vi "nanocal -- nuclear schottky fit V8.vi"() -> ()   [LabVIEW 2021] (continued)
 0.000000000000   ,  \"Reoff\" -> 0.000000000000   ,  \"Imoff\" -> 0.000000000000   ,  \"στ1\" -> 0.000000000000   ,  \"στS\" -> 0.000000000000   ,  \"στN\" -> 0.000000000000   ,  \"τ11 \" -> 0.000000000000   ,  \"τ12\" -> 0.000000000000   ,  \"τ22\" -> 0.000000000000   ,  \"τN1\" -> 0.000000000000   ,  \"τN2\" -> 0.000000000000   ,  \"σηlogτ1 \" -> 0.000000000000   ,  \"σηlogτS\" -> 0.000000000000   ,  \"σηlogτN\" -> 0.000000000000   ,  \"σlogτ1\" -> 0.000000000000   ,  \"σlogτS\" -> 0.000000000000   ,  \"σlogτN\" -> 0.000000000000   ,  \"σητ1\" -> 0.000000000000   ,  \"σητS \" -> 0.000000000000   ,  \"σητN\" -> 0.000000000000    |>   , \n\"IDS0168_210310_RAW_cal__ref_\" ->   <|    \"ζ\" -> 0.018175201883   ,  \"τ1\" -> 0.013383195137   ,  \"τS\" -> 0.017675939869   ,  \"τN\" -> 0.000584160710   ,  \"τC\" -> 0.005568397021   ,  \"κ0\" -> 0.000000005579   ,  \"mm1\" -> 0.000076155273   ,  \"mm2\" -> 0.012686054664   ,  \"mm3\" -> 0.024781363815   ,  \"T\" -> 0.810000000000   ,  \"B\" -> 12.000000000000   ,  \"θ\" -> 0.000000000000   ,  \"Reoff\" -> 0.000000000000   ,  \"Imoff\" -> 0.000000000000   ,  \"στ1\" -> 0.000105801087   ,  \"στS\" -> 0.000001832616   ,  \"στN\" -> 0.000002314917   ,  \"τ11 \" -> 0.000000000000   ,  \"τ12\" -> 0.000000000000   ,  \"τ22\" -> 0.000000000000   ,  \"τN1\" -> 0.000000000000   ,  \"τN2\" -> 0.000000000000   ,  \"σηlogτ1 \" -> 0.050518101739   ,  \"σηlogτS\" -> 0.000100664856   ,  \"σηlogτN\" -> 0.045919539288   ,  \"σlogτ1\" -> 0.007905517739   ,  \"σlogτS\" -> 0.000103678550   ,  \"σlogτN\" -> 0.003962808035   ,  \"σητ1\" -> 0.000676093614   ,  \"σητS \" -> 0.000001779346   ,  \"σητN\" -> 0.000026824391    |>   , \n\"IDS0168_210310_RAW_cal__sam_\" ->   <|    \"ζ\" -> 0.017558473054   ,  \"τ1\" -> 0.014545104284   ,  \"τS\" -> 0.022979681288   ,  \"τN\" -> 0.000840829385   ,  \"τC\" -> 0.005228030240   ,  \"κ0\" -> 0.000000006068   ,  \"mm1\" -> 0.000073916527   ,  \"mm2\" -> 0.013750428362   ,  \"mm3\" -> 0.030187552103   ,  \"T\" -> 0.810000000000   ,  \"B\" -> 12.000000000000   ,  \"θ\" -> 0.000000000000   ,  \"Reoff\" -> 0.000000000000   ,  \"Imoff\" -> 0.000000000000   ,  \"στ1\" -> 0.000000000000   ,  \"στS\" -> 0.000000000000   ,  \"στN\" -> 0.000000000000   ,  \"τ11 \" -> 0.000000000000   ,  \"τ12\" -> 0.000000000000   ,  \"τ22\" -> 0.000000000000   ,  \"τN1\" -> 0.000000000000   ,  \"τN2\" -> 0.000000000000   ,  \"σηlogτ1 \" -> 0.000000000000   ,  \"σηlogτS\" -> 0.000000000000   ,  \"σηlogτN\" -> 0.000000000000   ,  \"σlogτ1\" -> 0.000000000000   ,  \"σlogτS\" -> 0.000000000000   ,  \"σlogτN\" -> 0.000000000000   ,  \"σητ1\" -> 0.000000000000   ,  \"σητS \" -> 0.000000000000   ,  \"σητN\" -> 0.000000000000    |>   , \n\"IDS0169_210310_RAW_cal__ref_\" ->   <|    \"ζ\" -> 0.019957179421   ,  \"τ1\" -> 0.013979356395   ,  \"τS\" -> 0.014979933171   ,  \"τN\" -> 0.000246381668   ,  \"τC\" -> 0.003917957379   ,  \"κ0\" -> 0.000000007787   ,  \"mm1\" -> 0.000061209589   ,  \"mm2\" -> 0.013393834195   ,  \"mm3\" -> 0.019972459127   ,  \"T\" -> 1.120000000000   ,  \"B\" -> 12.000000000000   ,  \"θ\" -> 0.000000000000   ,  \"Reoff\" -> -604081.632653061067   ,  \"Imoff\" -> 0.000000000000   ,  \"στ1\" -> 0.016865078301   ,  \"στS\" -> 0.000159497722   ,  \"στN\" -> 0.007867947468   ,  \"τ11 \" -> 0.000000000000   ,  \"τ12\" -> 0.000000000000   ,  \"τ22\" -> 0.000000000000   ,  \"τN1\" -> 0.000000000000   ,  \"τN2\" -> 0.000000000000   ,  \"σηlogτ1 \" -> 0.000000000000   ,  \"σηlogτS\" -> 0.000000000000   ,  \"σηlogτN\" -> 0.000000000000   ,  \"σlogτ1\" -> 0.000000000000   ,  \"σlogτS\" -> 0.000000000000   ,  \"σlogτN\" -> 0.000000000000   ,  \"σητ1\" -> 0.000000000000   ,  \"σητS \" -> 0.000000000000   ,  \"σητN\" -> 0.000000000000    |>   , \n\"IDS0169_210310_RAW_cal__sam_\" ->   <|    \"ζ\" -> 0.011916480594   ,  \"τ1\" -> 0.012551282481   ,  \"τS\" -> 0.018233218660   ,  \"τN\" -> 0.000345702746   ,  \"τC\" -> 0.004699451527   ,  \"κ0\" -> 0.000000008451   ,  \"mm1\" -> 0.000044190864   ,  \"mm2\" -> 0.012162820727   ,  \"mm3\" -> 0.023844039179   ,  \"T\" -> 1.120000000000   ,  \"B\" -> 12.000000000000   ,  \"θ\" -> 0.000000000000   ,  \"Reoff\" -> 0.000000000000   ,  \"Imoff\" -> 0.000000000000   ,  \"στ1\" -> 0.000000000000   ,  \"στS\" -> 0.000000000000   ,  \"στN\" -> 0.000000000000   ,  \"τ11 \" -> 0.000000000000   ,  \"τ12\" -> 0.000000000000   ,  \"τ22\" -> 0.000000000000   ,  \"τN1\" -> 0.000000000000   ,  \"τN2\" -> 0.000000000000   ,  \"σηlogτ1 \" -> 0.000000000000   ,  \"σηlogτS\" -> 0.000000000000   ,  \"σηlogτN\" -> 0.000000000000   ,  \"σlogτ1\" -> 0.000000000000   ,  \"σlogτS\" -> 0.000000000000   ,  \"σlogτN\" -> 0.000000000000   ,  \"σητ1\" -> 0.000000000000   ,  \"σητS \" -> 0.000000000000   ,  \"σητN\" -> 0.000000000000    |>   , \n\"IDS0170_210310_RAW_cal__ref_\" ->   <|    \"ζ\" -> 0.020917521423   ,  \"τ1\" -> 0.014571936752   ,  \"τS\" -> 0.010774968577   ,  \"τN\" -> 0.000062073801   ,  \"τC\" -> 0.003888097391   ,  \"κ0\" -> 0.000000012613   ,  \"mm1\" -> 0.000059093319   ,  \"mm2\" -> 0.013758745196   ,  \"mm3\" -> 0.015705922073   ,  \"T\" -> 1.800000000000   ,  \"B\" -> 12.000000000000   ,  \"θ\" -> 0.000000000000   ,  \"Reoff\" -> -530612.244897959054   ,  \"Imoff\" -> 0.000000000000   ,  \"στ1\" -> 0.055735786157   ,  \"στS\" -> 0.000157216248   ,  \"στN\" -> 0.024225134913   ,  \"τ11 \" -> 0.000000000000   ,  \"τ12\" -> 0.000000000000   ,  \"τ22\" -> 0.000000000000   ,  \"τN1\" -> 0.000000000000   ,  \"τN2\" -> 0.000000000000   ,  \"σηlogτ1 \" -> 0.000000000000   ,  \"σηlogτS\" -> 0.000000000000   ,  \"σηlogτN\" -> 0.000000000000   ,  \"σlogτ1\" -> 0.000000000000   ,  \"σlogτS\" -> 0.000000000000   ,  \"σlogτN\" -> 0.000000000000   ,  \"σητ1\" -> 0.000000000000   ,  \"σητS \" -> 0.000000000000   ,  \"σητN\" -> 0.000000000000    |>   , \n\"IDS0170_210310_RAW_cal__sam_\" ->   <|    \"ζ\" -> 0.012831327568   ,  \"τ1\" -> 0.013315909415   ,  \"τS\" -> 0.012590836847   ,  \"τN\" -> 0.000065003013   ,  \"τC\" -> 0.005276356243   ,  \"κ0\" -> 0.000000013610   ,  \"mm1\" -> 0.000047406274   ,  \"mm2\" -> 0.013137605540   ,  \"mm3\" -> 0.018225484932   ,  \"T\" -> 1.800000000000   ,  \"B\" -> 12.000000000000   ,  \"θ\" -> 0.000000000000   ,  \"Reoff\" -> 0.000000000000   ,  \"Imoff\" -> 0.000000000000   ,  \"στ1\" -> 0.000000000000   ,  \"στS\" -> 0.000000000000   ,  \"στN\" -> 0.000000000000   ,  \"τ11 \" -> 0.000000000000   ,  \"τ12\" -> 0.000000000000   ,  \"τ22\" -> 0.000000000000   ,  \"τN1\" -> 0.000000000000   ,  \"τN2\" -> 0.000000000000   ,  \"σηlogτ1 \" -> 0.000000000000   ,  \"σηlogτS\" -> 0.000000000000   ,  \"σηlogτN\" -> 0.000000000000   ,  \"σlogτ1\" -> 0.000000000000   ,  \"σlogτS\" -> 0.000000000000   ,  \"σlogτN\" -> 0.000000000000   ,  \"σητ1\" -> 0.000000000000   ,  \"σητS \" -> 0.000000000000   ,  \"σητN\" -> 0.000000000000    |>   , \n\"IDS0171_210310_RAW_cal__ref_\" ->   <|    \"ζ\" -> 0.017116647721   ,  \"τ1\" -> 0.014941878219   ,  \"τS\" -> 0.008392436112   ,  \"τN\" -> 0.000011747084   ,  \"τC\" -> 0.002803142231   ,  \"κ0\" -> 0.000000022439   ,  \"mm1\" -> 0.000035623333   ,  \"mm2\" -> 0.011267010418   ,  \"mm3\" -> 0.014990421338   ,  \"T\" -> 3.100000000000   ,  \"B\" -> 12.000000000000   ,  \"θ\" -> 0.000000000000   ,  \"Reoff\" -> -297959.183673469349   ,  \"Imoff\" -> 0.000000000000   ,  \"στ1\" -> 0.410303910661   ,  \"στS\" -> 0.000232255759   ,  \"στN\" -> 0.188003802712   ,  \"τ11 \" -> 0.000000000000   ,  \"τ12\" -> 0.000000000000   ,  \"τ22\" -> 0.000000000000   ,  \"τN1\" -> 0.000000000000   ,  \"τN2\" -> 0.000000000000   ,  \"σηlogτ1 \" -> 0.000000000000   ,  \"σηlogτS\" -> 0.000000000000   ,  \"σηlogτN\" -> 0.000000000000   ,  \"σlogτ1\" -> 0.000000000000   ,  \"σlogτS\" -> 0.000000000000   ,  \"σlogτN\" -> 0.000000000000   ,  \"σητ1\" -> 0.000000000000   ,  \"σητS \" -> 0.000000000000   ,  \"σητN\" -> 0.000000000000    |>   , \n\"IDS0171_210310_RAW_cal__sam_\" ->   <|    \"ζ\" -> 0.019774146838   ,  \"τ1\" -> 0.013257273421   ,  \"τS\" -> 0.007064131508   ,  \"τN\" -> 0.000028000819   ,  \"τC\" -> 0.006942241845   ,  \"κ0\" -> 0.000000023477   ,  \"mm1\" -> 0.000068886863   ,  \"mm2\" -> 0.012935419574   ,  \"mm3\" -> 0.014427582022   ,  \"T\" -> 3.100000000000   ,  \"B\" -> 12.000000000000   ,  \"θ\" -> 0.000000000000   ,  \"Reoff\" -> 0.000000000000   ,  \"Imoff\" -> 0.000000000000   ,  \"στ1\" -> 0.000000000000   ,  \"στS\" -> 0.000000000000   ,  \"στN\" -> 0.000000000000   ,  \"τ11 \" -> 0.000000000000   ,  \"τ12\" -> 0.000000000000   ,  \"τ22\" -> 0.000000000000   ,  \"τN1\" -> 0.000000000000   ,  \"τN2\" -> 0.000000000000   ,  \"σηlogτ1 \" -> 0.000000000000   ,  \"σηlogτS\" -> 0.000000000000   ,  \"σηlogτN\" -> 0.000000000000   ,  \"σlogτ1\" -> 0.000000000000   ,  \"σlogτS\" -> 0.000000000000   ,  \"σlogτN\" -> 0.000000000000   ,  \"σητ1\" -> 0.000000000000   ,  \"σητS \" -> 0.000000000000   ,  \"σητN\" -> 0.000000000000    |>   , \n\"IDS0172_210310_RAW_cal__ref_\" ->   <|    \"ζ\" -> 0.018105234018   ,  \"τ1\" -> 0.013976020767   ,  \"τS\" -> 0.005494207082   ,  \"τN\" -> 0.000001697310   ,  \"τC\" -> 0.002434353238   ,  \"κ0\" -> 0.000000055294   ,  \"mm1\" -> 0.000030277813   ,  \"mm2\" -> 0.007995449956   ,  \"mm3\" -> 0.013980055263   ,  \"T\" -> 5.500000000000   ,  \"B\" -> 12.000000000000   ,  \"θ\" -> 0.000000000000   ,  \"Reoff\" -> -114285.714285714086   ,  \"Imoff\" -> 0.000000000000   ,  \"στ1\" -> 5.359406809289   ,  \"στS\" -> 0.000541837361   ,  \"στN\" -> 2.799281990955   ,  \"τ11 \" -> 0.000000000000   ,  \"τ12\" -> 0.000000000000   ,  \"τ22\" -> 0.000000000000   ,  \"τN1\" -> 0.000000000000   ,  \"τN2\" -> 0.000000000000   ,  \"σηlogτ1 \" -> 0.000000000000   ,  \"σηlogτS\" -> 0.000000000000   ,  \"σηlogτN\" -> 0.000000000000   ,  \"σlogτ1\" -> 0.000000000000   ,  \"σlogτS\" -> 0.000000000000   ,  \"σlogτN\" -> 0.000000000000   ,  \"σητ1\" -> 0.000000000000   ,  \"σητS \" -> 0.000000000000   ,  \"σητN\" -> 0.000000000000    |>   , \n\"IDS0172_210310_RAW_cal__sam_\" ->   <|    \"ζ\" -> 0.029251354442   ,  \"τ1\" -> 0.014634751206   ,  \"τS\" -> 0.003873958746   ,  \"τN\" -> 0.000007000487   ,  \"τC\" -> 0.006827504775   ,  \"κ0\" -> 0.000000056438   ,  \"mm1\" -> 0.000072018576   ,  \"mm2\" -> 0.010723236476   ,  \"mm3\" -> 0.014661483476   ,  \"T\" -> 5.500000000000   ,  \"B\" -> 12.000000000000   ,  \"θ\" -> 0.000000000000   ,  \"Reoff\" -> 0.000000000000   ,  \"Imoff\" -> 0.000000000000   ,  \"στ1\" -> 0.000000000000   ,  \"στS\" -> 0.000000000000   ,  \"στN\" -> 0.000000000000   ,  \"τ11 \" -> 0.000000000000   ,  \"τ12\" -> 0.000000000000   ,  \"τ22\" -> 0.000000000000   ,  \"τN1\" -> 0.000000000000   ,  \"τN2\" -> 0.000000000000   ,  \"σηlogτ1 \" -> 0.000000000000   ,  \"σηlogτS\" -> 0.000000000000   ,  \"σηlogτN\" -> 0.000000000000   ,  \"σlogτ1\" -> 0.000000000000   ,  \"σlogτS\" -> 0.000000000000   ,  \"σlogτN\" -> 0.000000000000   ,  \"σητ1\" -> 0.000000000000   ,  \"σητS \" -> 0.000000000000   ,  \"σητN\" -> 0.000000000000    |>   , \n\"IDS0181_210310_RAW_cal__ref_\" ->   <|    \"ζ\" -> 0.199306617611   ,  \"τ1\" -> 0.070107577087   ,  \"τS\" -> 0.034354681127   ,  \"τN\" -> 0.115326183519   ,  \"τC\" -> 0.001029913549   ,  \"κ0\" -> 0.000000000906   ,  \"mm1\" -> 0.000167619565   ,  \"mm2\" -> 0.012387908692   ,  \"mm3\" -> 0.238095213878   ,  \"T\" -> 0.179000000000   ,  \"B\" -> 12.000000000000   ,  \"θ\" -> 90.000000000000   ,  \"Reoff\" -> 0.000000000000   ,  \"Imoff\" -> 0.000000000000   ,  \"στ1\" -> 0.000080290810   ,  \"στS\" -> 0.000013361577   ,  \"στN\" -> 0.000100930245   ,  \"τ11 \" -> 0.000000000000   ,  \"τ12\" -> 0.000000000000   ,  \"τ22\" -> 0.000000000000   ,  \"τN1\" -> 0.000000000000   ,  \"τN2\" -> 0.000000000000   ,  \"σηlogτ1 \" -> 0.034187158287   ,  \"σηlogτS\" -> 0.001052177546   ,  \"σηlogτN\" -> 0.047354437967   ,  \"σlogτ1\" -> 0.001145251526   ,  \"σlogτS\" -> 0.000388930305   ,  \"σlogτN\" -> 0.000875171988   ,  \"σητ1\" -> 0.002396778835   ,  \"σητS \" -> 0.000036147224   ,  \"σητN\" -> 0.005461206603    |>   , \n\"IDS0181_210310_RAW_cal__sam_\" ->   <|    \"ζ\" -> 0.161975781729   ,  \"τ1\" -> 0.073089805113   ,  \"τS\" -> 0.045018408115   ,  \"τN\" -> 0.161987434028   ,  \"τC\" -> 0.001482104484   ,  \"κ0\" -> 0.000000001038   ,  \"mm1\" -> 0.000201615809   ,  \"mm2\" -> 0.012976126678   ,  \"mm3\" -> 0.301929942357   ,  \"T\" -> 0.179000000000   ,  \"B\" -> 12.000000000000   ,  \"θ\" -> 90.000000000000   ,  \"Reoff\" -> 0.000000000000   ,  \"Imoff\" -> 0.000000000000   ,  \"στ1\" -> 0.000000000000   ,  \"στS\" -> 0.000000000000   ,  \"στN\" -> 0.000000000000   ,  \"τ11 \" -> 0.000000000000   ,  \"τ12\" -> 0.000000000000   ,  \"τ22\" -> 0.000000000000   ,  \"τN1\" -> 0.000000000000   ,  \"τN2\" -> 0.000000000000   ,  \"σηlogτ1 \" -> 0.000000000000   ,  \"σηlogτS\" -> 0.000000000000   ,  \"σηlogτN\" -> 0.000000000000   ,  \"σlogτ1\" -> 0.000000000000   ,  \"σlogτS\" -> 0.000000000000   ,  \"σlogτN\" -> 0.000000000000   ,  \"σητ1\" -> 0.000000000000   ,  \"σητS \" -> 0.000000000000   ,  \"σητN\" -> 0.000000000000    |>   , \n\"IDS0183_210310_RAW_cal__ref_\" ->   <|    \"ζ\" -> 0.375235391174   ,  \"τ1\" -> 0.100390183494   ,  \"τS\" -> 0.059883674441   ,  \"τN\" -> 0.583268417564   ,  \"τC\" -> 0.001015388210   ,  \"κ0\" -> 0.000000000451   ,  \"mm1\" -> 0.000274513115   ,  \"mm2\" -> 0.008539722831   ,  \"mm3\" -> 0.977076854592   ,  \"T\" -> 0.120000000000   ,  \"B\" -> 12.000000000000   ,  \"θ\" -> 90.000000000000   ,  \"Reoff\" -> 0.000000000000   ,  \"Imoff\" -> 0.000000000000   ,  \"στ1\" -> 0.000375271363   ,  \"στS\" -> 0.000128650872   ,  \"στN\" -> 0.001598463820   ,  \"τ11 \" -> 0.000000000000   ,  \"τ12\" -> 0.000000000000   ,  \"τ22\" -> 0.000000000000   ,  \"τN1\" -> 0.000000000000   ,  \"τN2\" -> 0.000000000000   ,  \"σηlogτ1 \" -> 0.048375297950   ,  \"σηlogτS\" -> 0.002019546500   ,  \"σηlogτN\" -> 0.062171656813   ,  \"σlogτ1\" -> 0.003738128067   ,  \"σlogτS\" -> 0.002148346326   ,  \"σlogτN\" -> 0.002740528669   ,  \"σητ1\" -> 0.004856405038   ,  \"σητS \" -> 0.000120937865   ,  \"σητN\" -> 0.036262763887    |>   , \n\"IDS0183_210310_RAW_cal__sam_\" ->   <|    \"ζ\" -> 0.300863384227   ,  \"τ1\" -> 0.104924004009   ,  \"τS\" -> 0.071070599729   ,  \"τN\" -> 0.992887187112   ,  \"τC\" -> 0.001721587800   ,  \"κ0\" -> 0.000000000548   ,  \"mm1\" -> 0.000392216822   ,  \"mm2\" -> 0.006637384427   ,  \"mm3\" -> 1.483679717825   ,  \"T\" -> 0.120000000000   ,  \"B\" -> 12.000000000000   ,  \"θ\" -> 90.000000000000   ,  \"Reoff\" -> 0.000000000000   ,  \"Imoff\" -> 0.000000000000   ,  \"στ1\" -> 0.000000000000   ,  \"στS\" -> 0.000000000000   ,  \"στN\" -> 0.000000000000   ,  \"τ11 \" -> 0.000000000000   ,  \"τ12\" -> 0.000000000000   ,  \"τ22\" -> 0.000000000000   ,  \"τN1\" -> 0.000000000000   ,  \"τN2\" -> 0.000000000000   ,  \"σηlogτ1 \" -> 0.000000000000   ,  \"σηlogτS\" -> 0.000000000000   ,  \"σηlogτN\" -> 0.000000000000   ,  \"σlogτ1\" -> 0.000000000000   ,  \"σlogτS\" -> 0.000000000000   ,  \"σlogτN\" -> 0.000000000000   ,  \"σητ1\" -> 0.000000000000   ,  \"σητS \" -> 0.000000000000   ,  \"σητN\" -> 0.000000000000    |>   , \n\"IDS0184_210310_RAW_cal__ref_\" ->   <|    \"ζ\" -> 0.267189614091   ,  \"τ1\" -> 0.086925369127   ,  \"τS\" -> 0.044416499058   ,  \"τN\" -> 0.254096954422   ,  \"τC\" -> 0.000963914391   ,  \"κ0\" -> 0.000000000659   ,  \"mm1\" -> 0.000200487571   ,  \"mm2\" -> 0.010899085515   ,  \"mm3\" -> 0.455062858348   ,  \"T\" -> 0.148000000000   ,  \"B\" -> 12.000000000000   ,  \"θ\" -> 90.000000000000   ,  \"Reoff\" -> 0.000000000000   ,  \"Imoff\" -> 0.000000000000   ,  \"στ1\" -> 0.000162673595   ,  \"στS\" -> 0.000036959811   ,  \"στN\" -> 0.000362772077   ,  \"τ11 \" -> 0.000000000000   ,  \"τ12\" -> 0.000000000000   ,  \"τ22\" -> 0.000000000000   ,  \"τN1\" -> 0.000000000000   ,  \"τN2\" -> 0.000000000000   ,  \"σηlogτ1 \" -> 0.039106583663   ,  \"σηlogτS\" -> 0.001480745607   ,  \"σηlogτN\" -> 0.052582206660   ,  \"σlogτ1\" -> 0.001871416790   ,  \"σlogτS\" -> 0.000832118957   ,  \"σlogτN\" -> 0.001427691560   ,  \"σητ1\" -> 0.003399354220   ,  \"σητS \" -> 0.000065769536   ,  \"σητN\" -> 0.013360978569    |>   , \n\"IDS0184_210310_RAW_cal__sam_\" ->   <|    \"ζ\" -> 0.215697702358   ,  \"τ1\" -> 0.095971807771   ,  \"τS\" -> 0.069319630290   ,  \"τN\" -> 0.366712218878   ,  \"τC\" -> 0.001526252261   ,  \"κ0\" -> 0.000000000784   ,  \"mm1\" -> 0.000266752031   ,  \"mm2\" -> 0.013373263674   ,  \"mm3\" -> 0.613940961515   ,  \"T\" -> 0.148000000000   ,  \"B\" -> 12.000000000000   ,  \"θ\" -> 90.000000000000   ,  \"Reoff\" -> 0.000000000000   ,  \"Imoff\" -> 0.000000000000   ,  \"στ1\" -> 0.000000000000   ,  \"στS\" -> 0.000000000000   ,  \"στN\" -> 0.000000000000   ,  \"τ11 \" -> 0.000000000000   ,  \"τ12\" -> 0.000000000000   ,  \"τ22\" -> 0.000000000000   ,  \"τN1\" -> 0.000000000000   ,  \"τN2\" -> 0.000000000000   ,  \"σηlogτ1 \" -> 0.000000000000   ,  \"σηlogτS\" -> 0.000000000000   ,  \"σηlogτN\" -> 0.000000000000   ,  \"σlogτ1\" -> 0.000000000000   ,  \"σlogτS\" -> 0.000000000000   ,  \"σlogτN\" -> 0.000000000000   ,  \"σητ1\" -> 0.000000000000   ,  \"σητS \" -> 0.000000000000   ,  \"σητN\" -> 0.000000000000    |>   , \n\"IDS0185_210310_RAW_cal__ref_\" ->   <|    \"ζ\" -> 0.169435500052   ,  \"τ1\" -> 0.065522222520   ,  \"τS\" -> 0.031885966152   ,  \"τN\" -> 0.085736532349   ,  \"τC\" -> 0.001085511850   ,  \"κ0\" -> 0.000000001071   ,  \"mm1\" -> 0.000153416807   ,  \"mm2\" -> 0.013121484947   ,  \"mm3\" -> 0.190884757967   ,  \"T\" -> 0.197000000000   ,  \"B\" -> 12.000000000000   ,  \"θ\" -> 90.000000000000   ,  \"Reoff\" -> 0.000000000000   ,  \"Imoff\" -> 0.000000000000   ,  \"στ1\" -> 0.000057538627   ,  \"στS\" -> 0.000008322484   ,  \"στN\" -> 0.000057382706   ,  \"τ11 \" -> 0.000000000000   ,  \"τ12\" -> 0.000000000000   ,  \"τ22\" -> 0.000000000000   ,  \"τN1\" -> 0.000000000000   ,  \"τN2\" -> 0.000000000000   ,  \"σηlogτ1 \" -> 0.032785245148   ,  \"σηlogτS\" -> 0.000886609066   ,  \"σηlogτN\" -> 0.045894988103   ,  \"σlogτ1\" -> 0.000878154381   ,  \"σlogτS\" -> 0.000261007731   ,  \"σlogτN\" -> 0.000669291195   ,  \"σητ1\" -> 0.002148162128   ,  \"σητS \" -> 0.000028270387   ,  \"σητN\" -> 0.003934877132    |>   , \n\"IDS0185_210310_RAW_cal__sam_\" ->   <|    \"ζ\" -> 0.139117463690   ,  \"τ1\" -> 0.070330410174   ,  \"τS\" -> 0.040829719954   ,  \"τN\" -> 0.122434321115   ,  \"τC\" -> 0.001436112939   ,  \"κ0\" -> 0.000000001208   ,  \"mm1\" -> 0.000170710071   ,  \"mm2\" -> 0.013785404893   ,  \"mm3\" -> 0.243787328523   ,  \"T\" -> 0.197000000000   ,  \"B\" -> 12.000000000000   ,  \"θ\" -> 90.000000000000   ,  \"Reoff\" -> 0.000000000000   ,  \"Imoff\" -> 0.000000000000   ,  \"στ1\" -> 0.000000000000   ,  \"στS\" -> 0.000000000000   ,  \"στN\" -> 0.000000000000   ,  \"τ11 \" -> 0.000000000000   ,  \"τ12\" -> 0.000000000000   ,  \"τ22\" -> 0.000000000000   ,  \"τN1\" -> 0.000000000000   ,  \"τN2\" -> 0.000000000000   ,  \"σηlogτ1 \" -> 0.000000000000   ,  \"σηlogτS\" -> 0.000000000000   ,  \"σηlogτN\" -> 0.000000000000   ,  \"σlogτ1\" -> 0.000000000000   ,  \"σlogτS\" -> 0.000000000000   ,  \"σlogτN\" -> 0.000000000000   ,  \"σητ1\" -> 0.000000000000   ,  \"σητS \" -> 0.000000000000   ,  \"σητN\" -> 0.000000000000    |>   , \n\"IDS0186_210310_RAW_cal__ref_\" ->   <|    \"ζ\" -> 0.100232193660   ,  \"τ1\" -> 0.049981714900   ,  \"τS\" -> 0.026964705596   ,  \"τN\" -> 0.034498560244   ,  \"τC\" -> 0.001422553924   ,  \"κ0\" -> 0.000000001370   ,  \"mm1\" -> 0.000124145367   ,  \"mm2\" -> 0.014880634319   ,  \"mm3\" -> 0.104023352943   ,  \"T\" -> 0.249000000000   ,  \"B\" -> 12.000000000000   ,  \"θ\" -> 90.000000000000   ,  \"Reoff\" -> 0.000000000000   ,  \"Imoff\" -> 0.000000000000   ,  \"στ1\" -> 0.000091233173   ,  \"στS\" -> 0.000009463067   ,  \"στN\" -> 0.000045871847   ,  \"τ11 \" -> 0.000000000000   ,  \"τ12\" -> 0.000000000000   ,  \"τ22\" -> 0.000000000000   ,  \"τN1\" -> 0.000000000000   ,  \"τN2\" -> 0.000000000000   ,  \"σηlogτ1 \" -> 0.031503726160   ,  \"σηlogτS\" -> 0.000569534267   ,  \"σηlogτN\" -> 0.043675133431   ,  \"σlogτ1\" -> 0.001825330990   ,  \"σlogτS\" -> 0.000350942719   ,  \"σlogτN\" -> 0.001329674256   ,  \"σητ1\" -> 0.001574610259   ,  \"σητS \" -> 0.000015357324   ,  \"σητN\" -> 0.001506729222    |>   , \n\"IDS0186_210310_RAW_cal__sam_\" ->   <|    \"ζ\" -> 0.079912790251   ,  \"τ1\" -> 0.053932962768   ,  \"τS\" -> 0.033847624645   ,  \"τN\" -> 0.047947649984   ,  \"τC\" -> 0.001828917906   ,  \"κ0\" -> 0.000000001546   ,  \"mm1\" -> 0.000129305669   ,  \"mm2\" -> 0.016142481427   ,  \"mm3\" -> 0.127821856832   ,  \"T\" -> 0.249000000000   ,  \"B\" -> 12.000000000000   ,  \"θ\" -> 90.000000000000   ,  \"Reoff\" -> 0.000000000000   ,  \"Imoff\" -> 0.000000000000   ,  \"στ1\" -> 0.000000000000   ,  \"στS\" -> 0.000000000000   ,  \"στN\" -> 0.000000000000   ,  \"τ11 \" -> 0.000000000000   ,  \"τ12\" -> 0.000000000000   ,  \"τ22\" -> 0.000000000000   ,  \"τN1\" -> 0.000000000000   ,  \"τN2\" -> 0.000000000000   ,  \"σηlogτ1 \" -> 0.000000000000   ,  \"σηlogτS\" -> 0.000000000000   ,  \"σηlogτN\" -> 0.000000000000   ,  \"σlogτ1\" -> 0.000000000000   ,  \"σlogτS\" -> 0.000000000000   ,  \"σlogτN\" -> 0.000000000000   ,  \"σητ1\" -> 0.000000000000   ,  \"σητS \" -> 0.000000000000   ,  \"σητN\" -> 0.000000000000    |>   , \n\"IDS0187_210310_RAW_cal__ref_\" ->   <|    \"ζ\" -> 0.068889386962   ,  \"τ1\" -> 0.042189760597   ,  \"τS\" -> 0.023837806105   ,  \"τN\" -> 0.017176281362   ,  \"τC\" -> 0.001657645209   ,  \"κ0\" -> 0.000000001746   ,  \"mm1\" -> 0.000100672139   ,  \"mm2\" -> 0.015917651868   ,  \"mm3\" -> 0.071668604609   ,  \"T\" -> 0.300000000000   ,  \"B\" -> 12.000000000000   ,  \"θ\" -> 90.000000000000   ,  \"Reoff\" -> 0.000000000000   ,  \"Imoff\" -> 0.000000000000   ,  \"στ1\" -> 0.000071502532   ,  \"στS\" -> 0.000005082442   ,  \"στN\" -> 0.000020526312   ,  \"τ11 \" -> 0.000000000000   ,  \"τ12\" -> 0.000000000000   ,  \"τ22\" -> 0.000000000000   ,  \"τN1\" -> 0.000000000000   ,  \"τN2\" -> 0.000000000000   ,  \"σηlogτ1 \" -> 0.031154246719   ,  \"σηlogτS\" -> 0.000371188322   ,  \"σηlogτN\" -> 0.042807799707   ,  \"σlogτ1\" -> 0.001694784024   ,  \"σlogτS\" -> 0.000213209307   ,  \"σlogτN\" -> 0.001195038160   ,  \"σητ1\" -> 0.001314390211   ,  \"σητS \" -> 0.000008848315   ,  \"σητN\" -> 0.000735278812    |>   , \n\"IDS0187_210310_RAW_cal__sam_\" ->   <|    \"ζ\" -> 0.057938569833   ,  \"τ1\" -> 0.045244527663   ,  \"τS\" -> 0.029709028064   ,  \"τN\" -> 0.023577376257   ,  \"τC\" -> 0.002006607539   ,  \"κ0\" -> 0.000000001948   ,  \"mm1\" -> 0.000103608352   ,  \"mm2\" -> 0.017542867394   ,  \"mm3\" -> 0.085978401835   ,  \"T\" -> 0.300000000000   ,  \"B\" -> 12.000000000000   ,  \"θ\" -> 90.000000000000   ,  \"Reoff\" -> 0.000000000000   ,  \"Imoff\" -> 0.000000000000   ,  \"στ1\" -> 0.000000000000   ,  \"στS\" -> 0.000000000000   ,  \"στN\" -> 0.000000000000   ,  \"τ11 \" -> 0.000000000000   ,  \"τ12\" -> 0.000000000000   ,  \"τ22\" -> 0.000000000000   ,  \"τN1\" -> 0.000000000000   ,  \"τN2\" -> 0.000000000000   ,  \"σηlogτ1 \" -> 0.000000000000   ,  \"σηlogτS\" -> 0.000000000000   ,  \"σηlogτN\" -> 0.000000000000   ,  \"σlogτ1\" -> 0.000000000000   ,  \"σlogτS\" -> 0.000000000000   ,  \"σlogτN\" -> 0.000000000000   ,  \"σητ1\" -> 0.000000000000   ,  \"σητS \" -> 0.000000000000   ,  \"σητN\" -> 0.000000000000    |>   , \n\"IDS0188_210310_RAW_cal__ref_\" ->   <|    \"ζ\" -> 0.050855621628   ,  \"τ1\" -> 0.035114064267   ,  \"τS\" -> 0.021745076003   ,  \"τN\" -> 0.009940720882   ,  \"τC\" -> 0.002035754152   ,  \"κ0\" -> 0.000000002124   ,  \"mm1\" -> 0.000090783062   ,  \"mm2\" -> 0.016027821307   ,  \"mm3\" -> 0.054328411833   ,  \"T\" -> 0.360000000000   ,  \"B\" -> 12.000000000000   ,  \"θ\" -> 90.000000000000   ,  \"Reoff\" -> 0.000000000000   ,  \"Imoff\" -> 0.000000000000   ,  \"στ1\" -> 0.000051164040   ,  \"στS\" -> 0.000002904884   ,  \"στN\" -> 0.000009775078   ,  \"τ11 \" -> 0.000000000000   ,  \"τ12\" -> 0.000000000000   ,  \"τ22\" -> 0.000000000000   ,  \"τN1\" -> 0.000000000000   ,  \"τN2\" -> 0.000000000000   ,  \"σηlogτ1 \" -> 0.032086752475   ,  \"σηlogτS\" -> 0.000290620320   ,  \"σηlogτN\" -> 0.042734154502   ,  \"σlogτ1\" -> 0.001457081108   ,  \"σlogτS\" -> 0.000133588143   ,  \"σlogτN\" -> 0.000983336979   ,  \"σητ1\" -> 0.001126696289   ,  \"σητS \" -> 0.000006319561   ,  \"σητN\" -> 0.000424808302    |>   , \n\"IDS0188_210310_RAW_cal__sam_\" ->   <|    \"ζ\" -> 0.044154556051   ,  \"τ1\" -> 0.038823125235   ,  \"τS\" -> 0.027069314930   ,  \"τN\" -> 0.013601990730   ,  \"τC\" -> 0.002287979276   ,  \"κ0\" -> 0.000000002359   ,  \"mm1\" -> 0.000089763345   ,  \"mm2\" -> 0.018083678254   ,  \"mm3\" -> 0.065404792018   ,  \"T\" -> 0.360000000000   ,  \"B\" -> 12.000000000000   ,  \"θ\" -> 90.000000000000   ,  \"Reoff\" -> 0.000000000000   ,  \"Imoff\" -> 0.000000000000   ,  \"στ1\" -> 0.000000000000   ,  \"στS\" -> 0.000000000000   ,  \"στN\" -> 0.000000000000   ,  \"τ11 \" -> 0.000000000000   ,  \"τ12\" -> 0.000000000000   ,  \"τ22\" -> 0.000000000000   ,  \"τN1\" -> 0.000000000000   ,  \"τN2\" -> 0.000000000000   ,  \"σηlogτ1 \" -> 0.000000000000   ,  \"σηlogτS\" -> 0.000000000000   ,  \"σηlogτN\" -> 0.000000000000   ,  \"σlogτ1\" -> 0.000000000000   ,  \"σlogτS\" -> 0.000000000000   ,  \"σlogτN\" -> 0.000000000000   ,  \"σητ1\" -> 0.000000000000   ,  \"σητS \" -> 0.000000000000   ,  \"σητN\" -> 0.000000000000    |>   , \n\"IDS0189_210310_RAW_cal__ref_\" ->   <|    \"ζ\" -> 0.038379394547   ,  \"τ1\" -> 0.030049345911   ,  \"τS\" -> 0.020197203084   ,  \"τN\" -> 0.005279271749   ,  \"τC\" -> 0.002296433055   ,  \"κ0\" -> 0.000000002676   ,  \"mm1\" -> 0.000076749631   ,  \"mm2\" -> 0.016510358322   ,  \"mm3\" -> 0.042212917525   ,  \"T\" -> 0.430000000000   ,  \"B\" -> 12.000000000000   ,  \"θ\" -> 90.000000000000   ,  \"Reoff\" -> 0.000000000000   ,  \"Imoff\" -> 0.000000000000   ,  \"στ1\" -> 0.000059898317   ,  \"στS\" -> 0.000002370734   ,  \"στN\" -> 0.000006802565   ,  \"τ11 \" -> 0.000000000000   ,  \"τ12\" -> 0.000000000000   ,  \"τ22\" -> 0.000000000000   ,  \"τN1\" -> 0.000000000000   ,  \"τN2\" -> 0.000000000000   ,  \"σηlogτ1 \" -> 0.033097505686   ,  \"σηlogτS\" -> 0.000200297015   ,  \"σηlogτN\" -> 0.042720953668   ,  \"σlogτ1\" -> 0.001993331815   ,  \"σlogτS\" -> 0.000117379325   ,  \"σlogτN\" -> 0.001288542279   ,  \"σητ1\" -> 0.000994558397   ,  \"σητS \" -> 0.000004045439   ,  \"σητN\" -> 0.000225535524    |>   , \n\"IDS0189_210310_RAW_cal__sam_\" ->   <|    \"ζ\" -> 0.032748569996   ,  \"τ1\" -> 0.031072007290   ,  \"τS\" -> 0.024343937548   ,  \"τN\" -> 0.006961654481   ,  \"τC\" -> 0.002967111565   ,  \"κ0\" -> 0.000000002964   ,  \"mm1\" -> 0.000084402249   ,  \"mm2\" -> 0.018055855929   ,  \"mm3\" -> 0.048229666078   ,  \"T\" -> 0.430000000000   ,  \"B\" -> 12.000000000000   ,  \"θ\" -> 90.000000000000   ,  \"Reoff\" -> 0.000000000000   ,  \"Imoff\" -> 0.000000000000   ,  \"στ1\" -> 0.000000000000   ,  \"στS\" -> 0.000000000000   ,  \"στN\" -> 0.000000000000   ,  \"τ11 \" -> 0.000000000000   ,  \"τ12\" -> 0.000000000000   ,  \"τ22\" -> 0.000000000000   ,  \"τN1\" -> 0.000000000000   ,  \"τN2\" -> 0.000000000000   ,  \"σηlogτ1 \" -> 0.000000000000   ,  \"σηlogτS\" -> 0.000000000000   ,  \"σηlogτN\" -> 0.000000000000   ,  \"σlogτ1\" -> 0.000000000000   ,  \"σlogτS\" -> 0.000000000000   ,  \"σlogτN\" -> 0.000000000000   ,  \"σητ1\" -> 0.000000000000   ,  \"σητS \" -> 0.000000000000   ,  \"σητN\" -> 0.000000000000    |>   , \n\"IDS0190_210310_RAW_cal__ref_\" ->   <|    \"ζ\" -> 0.030757711173   ,  \"τ1\" -> 0.024931554661   ,  \"τS\" -> 0.019059366283   ,  \"τN\" -> 0.002804912424   ,  \"τC\" -> 0.002400955690   ,  \"κ0\" -> 0.000000003344   ,  \"mm1\" -> 0.000064025305   ,  \"mm2\" -> 0.016413784329   ,  \"mm3\" -> 0.033391474593   ,  \"T\" -> 0.512000000000   ,  \"B\" -> 12.000000000000   ,  \"θ\" -> 90.000000000000   ,  \"Reoff\" -> 0.000000000000   ,  \"Imoff\" -> 0.000000000000   ,  \"στ1\" -> 0.000088127283   ,  \"στS\" -> 0.000002533160   ,  \"στN\" -> 0.000006068263   ,  \"τ11 \" -> 0.000000000000   ,  \"τ12\" -> 0.000000000000   ,  \"τ22\" -> 0.000000000000   ,  \"τN1\" -> 0.000000000000   ,  \"τN2\" -> 0.000000000000   ,  \"σηlogτ1 \" -> 0.035038614150   ,  \"σηlogτS\" -> 0.000144373831   ,  \"σηlogτN\" -> 0.043033459724   ,  \"σlogτ1\" -> 0.003534768852   ,  \"σlogτS\" -> 0.000132908910   ,  \"σlogτN\" -> 0.002163441144   ,  \"σητ1\" -> 0.000873567124   ,  \"σητS \" -> 0.000002751674   ,  \"σητN\" -> 0.000120705086    |>   , \n\"IDS0190_210310_RAW_cal__sam_\" ->   <|    \"ζ\" -> 0.027599263457   ,  \"τ1\" -> 0.026239105728   ,  \"τS\" -> 0.022370859308   ,  \"τN\" -> 0.003857632966   ,  \"τC\" -> 0.003499360499   ,  \"κ0\" -> 0.000000003681   ,  \"mm1\" -> 0.000081816106   ,  \"mm2\" -> 0.017901054668   ,  \"mm3\" -> 0.038707974796   ,  \"T\" -> 0.512000000000   ,  \"B\" -> 12.000000000000   ,  \"θ\" -> 90.000000000000   ,  \"Reoff\" -> 0.000000000000   ,  \"Imoff\" -> 0.000000000000   ,  \"στ1\" -> 0.000000000000   ,  \"στS\" -> 0.000000000000   ,  \"στN\" -> 0.000000000000   ,  \"τ11 \" -> 0.000000000000   ,  \"τ12\" -> 0.000000000000   ,  \"τ22\" -> 0.000000000000   ,  \"τN1\" -> 0.000000000000   ,  \"τN2\" -> 0.000000000000   ,  \"σηlogτ1 \" -> 0.000000000000   ,  \"σηlogτS\" -> 0.000000000000   ,  \"σηlogτN\" -> 0.000000000000   ,  \"σlogτ1\" -> 0.000000000000   ,  \"σlogτS\" -> 0.000000000000   ,  \"σlogτN\" -> 0.000000000000   ,  \"σητ1\" -> 0.000000000000   ,  \"σητS \" -> 0.000000000000   ,  \"σητN\" -> 0.000000000000    |>   , \n\"IDS0191_210310_RAW_cal__ref_\" ->   <|    \"ζ\" -> 0.024472356387   ,  \"τ1\" -> 0.022407083343   ,  \"τS\" -> 0.017600386438   ,  \"τN\" -> 0.001730254025   ,  \"τC\" -> 0.003444856237   ,  \"κ0\" -> 0.000000003989   ,  \"mm1\" -> 0.000069310557   ,  \"mm2\" -> 0.016480900420   ,  \"mm3\" -> 0.029105435389   ,  \"T\" -> 0.610000000000   ,  \"B\" -> 12.000000000000   ,  \"θ\" -> 90.000000000000   ,  \"Reoff\" -> 0.000000000000   ,  \"Imoff\" -> 0.000000000000   ,  \"στ1\" -> 0.000087154359   ,  \"στS\" -> 0.000001846195   ,  \"στN\" -> 0.000003983538   ,  \"τ11 \" -> 0.000000000000   ,  \"τ12\" -> 0.000000000000   ,  \"τ22\" -> 0.000000000000   ,  \"τN1\" -> 0.000000000000   ,  \"τN2\" -> 0.000000000000   ,  \"σηlogτ1 \" -> 0.036359774839   ,  \"σηlogτS\" -> 0.000111954983   ,  \"σηlogτN\" -> 0.043247347257   ,  \"σlogτ1\" -> 0.003889589636   ,  \"σlogτS\" -> 0.000104895132   ,  \"σlogτN\" -> 0.002302284973   ,  \"σητ1\" -> 0.000814716505   ,  \"σητS \" -> 0.000001970451   ,  \"σητN\" -> 0.000074828897    |>   , \n\"IDS0191_210310_RAW_cal__sam_\" ->   <|    \"ζ\" -> 0.020568815513   ,  \"τ1\" -> 0.023045965648   ,  \"τS\" -> 0.020791387386   ,  \"τN\" -> 0.002229171297   ,  \"τC\" -> 0.004427475438   ,  \"κ0\" -> 0.000000004398   ,  \"mm1\" -> 0.000074037290   ,  \"mm2\" -> 0.017820522459   ,  \"mm3\" -> 0.033072945644   ,  \"T\" -> 0.610000000000   ,  \"B\" -> 12.000000000000   ,  \"θ\" -> 90.000000000000   ,  \"Reoff\" -> 0.000000000000   ,  \"Imoff\" -> 0.000000000000   ,  \"στ1\" -> 0.000000000000   ,  \"στS\" -> 0.000000000000   ,  \"στN\" -> 0.000000000000   ,  \"τ11 \" -> 0.000000000000   ,  \"τ12\" -> 0.000000000000   ,  \"τ22\" -> 0.000000000000   ,  \"τN1\" -> 0.000000000000   ,  \"τN2\" -> 0.000000000000   ,  \"σηlogτ1 \" -> 0.000000000000   ,  \"σηlogτS\" -> 0.000000000000   ,  \"σηlogτN\" -> 0.000000000000   ,  \"σlogτ1\" -> 0.000000000000   ,  \"σlogτS\" -> 0.000000000000   ,  \"σlogτN\" -> 0.000000000000   ,  \"σητ1\" -> 0.000000000000   ,  \"σητS \" -> 0.000000000000   ,  \"σητN\" -> 0.000000000000    |>   , \n\"IDS0192_210310_RAW_cal__ref_\" ->   <|    \"ζ\" -> 0.019125590894   ,  \"τ1\" -> 0.016432131318   ,  \"τS\" -> 0.016139955363   ,  \"τN\" -> 0.000695948251   ,  \"τC\" -> 0.003787605771   ,  \"κ0\" -> 0.000000005582   ,  \"mm1\" -> 0.000057940868   ,  \"mm2\" -> 0.014584556611   ,  \"mm3\" -> 0.022735139829   ,  \"T\" -> 0.810000000000   ,  \"B\" -> 12.000000000000   ,  \"θ\" -> 90.000000000000   ,  \"Reoff\" -> 0.000000000000   ,  \"Imoff\" -> 0.000000000000   ,  \"στ1\" -> 0.000129667374   ,  \"στS\" -> 0.000001793381   ,  \"στN\" -> 0.000002982571   ,  \"τ11 \" -> 0.000000000000   ,  \"τ12\" -> 0.000000000000   ,  \"τ22\" -> 0.000000000000   ,  \"τN1\" -> 0.000000000000   ,  \"τN2\" -> 0.000000000000   ,  \"σηlogτ1 \" -> 0.041303896436   ,  \"σηlogτS\" -> 0.000075013998   ,  \"σηlogτN\" -> 0.044217367932   ,  \"σlogτ1\" -> 0.007891086787   ,  \"σlogτS\" -> 0.000111114402   ,  \"σlogτN\" -> 0.004285622428   ,  \"σητ1\" -> 0.000678711050   ,  \"σητS \" -> 0.000001210723   ,  \"σητN\" -> 0.000030773000    |>   , \n\"IDS0192_210310_RAW_cal__sam_\" ->   <|    \"ζ\" -> 0.016548170999   ,  \"τ1\" -> 0.020108887890   ,  \"τS\" -> 0.018558394948   ,  \"τN\" -> 0.001160732495   ,  \"τC\" -> 0.004746126241   ,  \"κ0\" -> 0.000000005882   ,  \"mm1\" -> 0.000061890920   ,  \"mm2\" -> 0.017029753868   ,  \"mm3\" -> 0.027808812278   ,  \"T\" -> 0.810000000000   ,  \"B\" -> 12.000000000000   ,  \"θ\" -> 90.000000000000   ,  \"Reoff\" -> 0.000000000000   ,  \"Imoff\" -> 0.000000000000   ,  \"στ1\" -> 0.000000000000   ,  \"στS\" -> 0.000000000000   ,  \"στN\" -> 0.000000000000   ,  \"τ11 \" -> 0.000000000000   ,  \"τ12\" -> 0.000000000000   ,  \"τ22\" -> 0.000000000000   ,  \"τN1\" -> 0.000000000000   ,  \"τN2\" -> 0.000000000000   ,  \"σηlogτ1 \" -> 0.000000000000   ,  \"σηlogτS\" -> 0.000000000000   ,  \"σηlogτN\" -> 0.000000000000   ,  \"σlogτ1\" -> 0.000000000000   ,  \"σlogτS\" -> 0.000000000000   ,  \"σlogτN\" -> 0.000000000000   ,  \"σητ1\" -> 0.000000000000   ,  \"σητS \" -> 0.000000000000   ,  \"σητN\" -> 0.000000000000    |>   , \n\"IDS0193_210310_RAW_cal__ref_\" ->   <|    \"ζ\" -> 0.016340595254   ,  \"τ1\" -> 0.016915232020   ,  \"τS\" -> 0.015114072822   ,  \"τN\" -> 0.000265648688   ,  \"τC\" -> 0.003610389555   ,  \"κ0\" -> 0.000000007797   ,  \"mm1\" -> 0.000047117169   ,  \"mm2\" -> 0.015633505106   ,  \"mm3\" -> 0.020476034614   ,  \"T\" -> 1.100000000000   ,  \"B\" -> 12.000000000000   ,  \"θ\" -> 90.000000000000   ,  \"Reoff\" -> 0.000000000000   ,  \"Imoff\" -> 0.000000000000   ,  \"στ1\" -> 0.000367130935   ,  \"στS\" -> 0.000001790268   ,  \"στN\" -> 0.000003209434   ,  \"τ11 \" -> 0.000000000000   ,  \"τ12\" -> 0.000000000000   ,  \"τ22\" -> 0.000000000000   ,  \"τN1\" -> 0.000000000000   ,  \"τN2\" -> 0.000000000000   ,  \"σηlogτ1 \" -> 0.039284134925   ,  \"σηlogτS\" -> 0.000026409322   ,  \"σηlogτN\" -> 0.043727840988   ,  \"σlogτ1\" -> 0.021704161954   ,  \"σlogτS\" -> 0.000118450384   ,  \"σlogτN\" -> 0.012081499151   ,  \"σητ1\" -> 0.000664500257   ,  \"σητS \" -> 0.000000399152   ,  \"σητN\" -> 0.000011616244    |>   , \n\"IDS0193_210310_RAW_cal__sam_\" ->   <|    \"ζ\" -> 0.014495870556   ,  \"τ1\" -> 0.019990087457   ,  \"τS\" -> 0.016832201384   ,  \"τN\" -> 0.000455517238   ,  \"τC\" -> 0.005555782498   ,  \"κ0\" -> 0.000000008420   ,  \"mm1\" -> 0.000060055560   ,  \"mm2\" -> 0.018114231010   ,  \"mm3\" -> 0.024909902538   ,  \"T\" -> 1.100000000000   ,  \"B\" -> 12.000000000000   ,  \"θ\" -> 90.000000000000   ,  \"Reoff\" -> 0.000000000000   ,  \"Imoff\" -> 0.000000000000   ,  \"στ1\" -> 0.000000000000   ,  \"στS\" -> 0.000000000000   ,  \"στN\" -> 0.000000000000   ,  \"τ11 \" -> 0.000000000000   ,  \"τ12\" -> 0.000000000000   ,  \"τ22\" -> 0.000000000000   ,  \"τN1\" -> 0.000000000000   ,  \"τN2\" -> 0.000000000000   ,  \"σηlogτ1 \" -> 0.000000000000   ,  \"σηlogτS\" -> 0.000000000000   ,  \"σηlogτN\" -> 0.000000000000   ,  \"σlogτ1\" -> 0.000000000000   ,  \"σlogτS\" -> 0.000000000000   ,  \"σlogτN\" -> 0.000000000000   ,  \"σητ1\" -> 0.000000000000   ,  \"σητS \" -> 0.000000000000   ,  \"σητN\" -> 0.000000000000    |>   , \n\"IDS0194_210310_RAW_cal__ref_\" ->   <|    \"ζ\" -> 0.012634392580   ,  \"τ1\" -> 0.012311180561   ,  \"τS\" -> 0.011880374999   ,  \"τN\" -> 0.000066834392   ,  \"τC\" -> 0.004093585380   ,  \"κ0\" -> 0.000000013452   ,  \"mm1\" -> 0.000038198127   ,  \"mm2\" -> 0.012105563906   ,  \"mm3\" -> 0.016359159033   ,  \"T\" -> 1.800000000000   ,  \"B\" -> 12.000000000000   ,  \"θ\" -> 90.000000000000   ,  \"Reoff\" -> 0.000000000000   ,  \"Imoff\" -> 0.000000000000   ,  \"στ1\" -> 0.000860954265   ,  \"στS\" -> 0.000001598192   ,  \"στN\" -> 0.000002482039   ,  \"τ11 \" -> 0.000000000000   ,  \"τ12\" -> 0.000000000000   ,  \"τ22\" -> 0.000000000000   ,  \"τN1\" -> 0.000000000000   ,  \"τN2\" -> 0.000000000000   ,  \"σηlogτ1 \" -> 0.042675275628   ,  \"σηlogτS\" -> 0.000010894575   ,  \"σηlogτN\" -> 0.044389870063   ,  \"σlogτ1\" -> 0.069932713660   ,  \"σlogτS\" -> 0.000134523688   ,  \"σlogτN\" -> 0.037137152263   ,  \"σητ1\" -> 0.000525383024   ,  \"σητS \" -> 0.000000129432   ,  \"σητN\" -> 0.000002966770    |>   , \n\"IDS0194_210310_RAW_cal__sam_\" ->   <|    \"ζ\" -> 0.014043763709   ,  \"τ1\" -> 0.018292068543   ,  \"τS\" -> 0.011311396743   ,  \"τN\" -> 0.000128802259   ,  \"τC\" -> 0.008087849636   ,  \"κ0\" -> 0.000000014258   ,  \"mm1\" -> 0.000065912054   ,  \"mm2\" -> 0.017276417784   ,  \"mm3\" -> 0.020638450794   ,  \"T\" -> 1.800000000000   ,  \"B\" -> 12.000000000000   ,  \"θ\" -> 90.000000000000   ,  \"Reoff\" -> 0.000000000000   ,  \"Imoff\" -> 0.000000000000   ,  \"στ1\" -> 0.000000000000   ,  \"στS\" -> 0.000000000000   ,  \"στN\" -> 0.000000000000   ,  \"τ11 \" -> 0.000000000000   ,  \"τ12\" -> 0.000000000000   ,  \"τ22\" -> 0.000000000000   ,  \"τN1\" -> 0.000000000000   ,  \"τN2\" -> 0.000000000000   ,  \"σηlogτ1 \" -> 0.000000000000   ,  \"σηlogτS\" -> 0.000000000000   ,  \"σηlogτN\" -> 0.000000000000   ,  \"σlogτ1\" -> 0.000000000000   ,  \"σlogτS\" -> 0.000000000000   ,  \"σlogτN\" -> 0.000000000000   ,  \"σητ1\" -> 0.000000000000   ,  \"σητS \" -> 0.000000000000   ,  \"σητN\" -> 0.000000000000    |>   , \n\"IDS0195_210310_RAW_cal__ref_\" ->   <|    \"ζ\" -> 0.019026086981   ,  \"τ1\" -> 0.018297259133   ,  \"τS\" -> 0.007367031681   ,  \"τN\" -> 0.000012328467   ,  \"τC\" -> 0.005085235141   ,  \"κ0\" -> 0.000000023922   ,  \"mm1\" -> 0.000056860147   ,  \"mm2\" -> 0.012508508795   ,  \"mm3\" -> 0.018336885828   ,  \"T\" -> 3.000000000000   ,  \"B\" -> 12.000000000000   ,  \"θ\" -> 90.000000000000   ,  \"Reoff\" -> -126530.612244897755   ,  \"Imoff\" -> 0.000000000000   ,  \"στ1\" -> 0.473735460179   ,  \"στS\" -> 0.000298320672   ,  \"στN\" -> 0.226260580227   ,  \"τ11 \" -> 0.000000000000   ,  \"τ12\" -> 0.000000000000   ,  \"τ22\" -> 0.000000000000   ,  \"τN1\" -> 0.000000000000   ,  \"τN2\" -> 0.000000000000   ,  \"σηlogτ1 \" -> 0.000000000000   ,  \"σηlogτS\" -> 0.000000000000   ,  \"σηlogτN\" -> 0.000000000000   ,  \"σlogτ1\" -> 0.000000000000   ,  \"σlogτS\" -> 0.000000000000   ,  \"σlogτN\" -> 0.000000000000   ,  \"σητ1\" -> 0.000000000000   ,  \"σητS \" -> 0.000000000000   ,  \"σητN\" -> 0.000000000000    |>   , \n\"IDS0195_210310_RAW_cal__sam_\" ->   <|    \"ζ\" -> 0.016187684631   ,  \"τ1\" -> 0.018325345271   ,  \"τS\" -> 0.007510087776   ,  \"τN\" -> 0.000028419157   ,  \"τC\" -> 0.008115463080   ,  \"κ0\" -> 0.000000024747   ,  \"mm1\" -> 0.000062903858   ,  \"mm2\" -> 0.015524812312   ,  \"mm3\" -> 0.018513630087   ,  \"T\" -> 3.000000000000   ,  \"B\" -> 12.000000000000   ,  \"θ\" -> 90.000000000000   ,  \"Reoff\" -> 0.000000000000   ,  \"Imoff\" -> 0.000000000000   ,  \"στ1\" -> 0.000000000000   ,  \"στS\" -> 0.000000000000   ,  \"στN\" -> 0.000000000000   ,  \"τ11 \" -> 0.000000000000   ,  \"τ12\" -> 0.000000000000   ,  \"τ22\" -> 0.000000000000   ,  \"τN1\" -> 0.000000000000   ,  \"τN2\" -> 0.000000000000   ,  \"σηlogτ1 \" -> 0.000000000000   ,  \"σηlogτS\" -> 0.000000000000   ,  \"σηlogτN\" -> 0.000000000000   ,  \"σlogτ1\" -> 0.000000000000   ,  \"σlogτS\" -> 0.000000000000   ,  \"σlogτN\" -> 0.000000000000   ,  \"σητ1\" -> 0.000000000000   ,  \"σητS \" -> 0.000000000000   ,  \"σητN\" -> 0.000000000000    |>   , \n\"IDS0196_210310_RAW_cal__ref_\" ->   <|    \"ζ\" -> 0.019858524497   ,  \"τ1\" -> 0.012821278093   ,  \"τS\" -> 0.004631070276   ,  
